vi "Check-acceleration.vi"(8 "error in (no error)":errorcluster, 10 "Acceleration in":dbl, 11 "Motor-Maxon in":refnum<class "Motor-Maxon.lvclass">) -> (0 "error out":errorcluster, 1 "In range?":bool, 2 "Acceleration out":dbl, 3 "Motor-Maxon out":refnum<class "Motor-Maxon.lvclass">)   [LabVIEW 2013, in "PowderDeposition.lvlib" / "Motor-Maxon.lvclass"]
uses:
  Motor-Maxon.lvclass
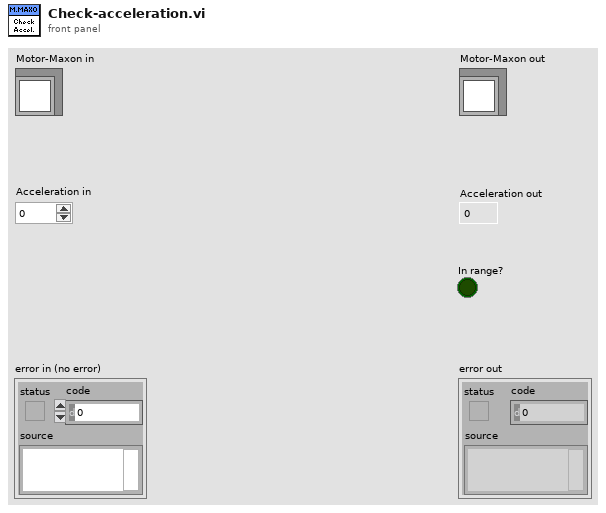
[diagram p1: front panel]
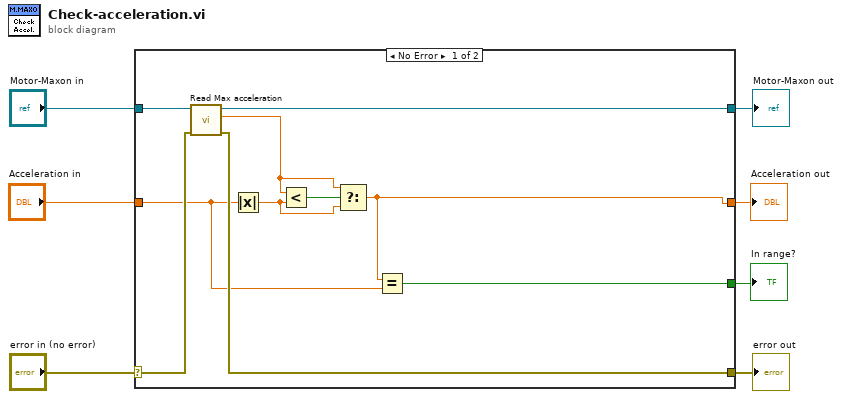
[diagram p0: block diagram]
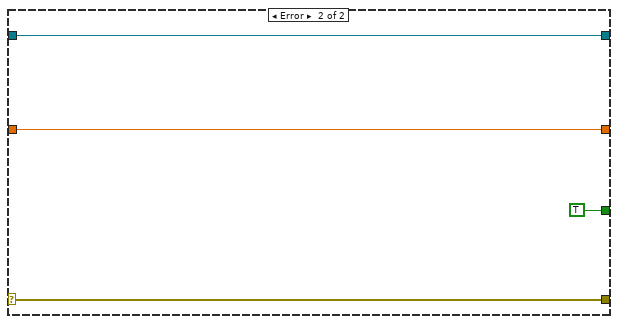
[diagram p2: hidden frame]
diagram:
  n1 = case shown="No Error" "error in (no error)" {
    selector: "error in (no error)" -> [w15 w21]
    tunnel: [w14 w21] -> w6
    tunnel: [w16 w20] -> w4
    tunnel: "Motor-Maxon in" -> [w17 w20]
    tunnel: "Acceleration in" -> [w10 w19]
    tunnel: [w8 w19] -> w2
    tunnel: [w9 TRUE] -> w1
    frame No Error {
      n2 = call-dynamic "Read Max acceleration.vi"("error in (no error)"=w15, "Motor-Maxon in"=w17) -> ("error out"=w14:errorcluster, "Max acceleration"=w12:dbl, "Motor-Maxon out"=w16:refnum<class "Motor-Maxon.lvclass">)  [unwired: 7 in]
      n3 = Absolute Value(x=w10) -> (abs(x)=w11:dbl)
      n4 = Less?(x=w12, y=w11) -> (x < y?=w13:bool)
      n5 = Select(t=w12, s=w13, f=w11) -> (s? t:f=w8:dbl)
      n6 = Equal?(x=w8, y=w10) -> (x = y?=w9:bool)
    }
    frame Error {
    }
  }
  "error out" <- w6
  "Motor-Maxon out" <- w4
  "Acceleration out" <- w2
  "In range?" <- w1
